vi "open.vi"(0 "object in":refnum<class "MBinteractive.lvclass">, 5 "error in (no error)":errorcluster) -> (14 "object out":refnum<class "MBinteractive.lvclass">, 19 "error out":errorcluster)   [LabVIEW 2016, in "MBinteractive.lvclass"]
uses:
  MBinteractive.lvclass
  <vilib>/NI/Modbus Library/API/Modbus API.lvclass/Modbus API.ctl
  <vilib>/NI/Modbus Library/Transmission Data Unit/Transmission Data Unit.lvclass/Transmission Data Unit.ctl
  MBinteractive.lvclass/MBinteractive.ctl
  <vilib>/NI/Modbus Library/API/Master/Set Unit ID.vi
  <vilib>/NI/Modbus Library/Transmission Data Unit/Write Unit ID.vi
  <vilib>/NI/Modbus Library/API/Read Transmission Data Unit.vi
  <vilib>/NI/Modbus Library/API/Write Transmission Data Unit.vi
  <vilib>/NI/Modbus Library/API/master/Modbus Master.lvclass
  D:/Program Files (x86)/National Instruments/LabVIEW 2016/vi.lib/NI/Modbus Library/API/Modbus API.lvclass
  <vilib>/NI/Modbus Library/API/Wrapper/Create TCP Master.vi
  <vilib>/NI/Modbus Library/API/Wrapper/API Main.lvlib
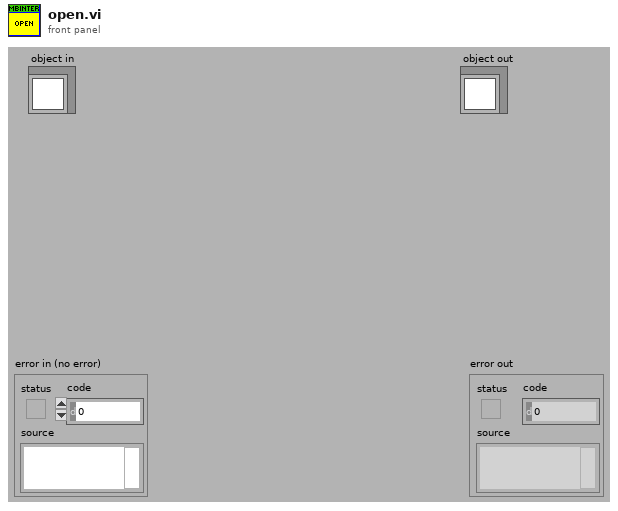
[diagram p1: front panel]
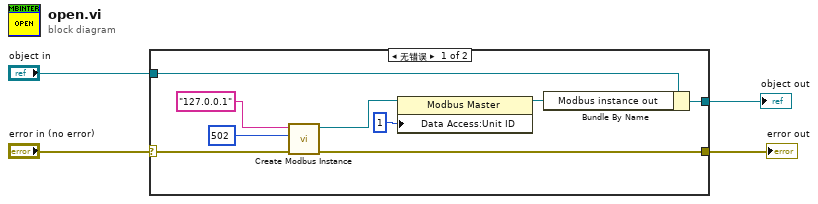
[diagram p0: block diagram]
diagram:
  n1 = case shown="无错误" "error in (no error)" {
    selector: "error in (no error)" -> [w6 w15]
    tunnel: [w5 w15] -> w3
    tunnel: [w12 w14] -> w1
    tunnel: "object in" -> [w13 w14]
    frame No Error {
      n2 = call-poly <vilib>:"Create Modbus Instance.vi"("error in"=w6, "port (502)"=u16 502, "address"="127.0.0.1") -> ("error out"=w5:errorcluster, "TCP master instance"=w11:refnum<class "Modbus Master.lvclass">)  [unwired: 7 in]
      n3 = property class="Modbus Master"(reference=w11, "Data Access:Unit ID"=u8 1 ("Unit ID")) -> (reference out=w7:refnum<class "Modbus Master.lvclass">)  [unwired: 1 in, 1 out]
      n4 = Bundle By Name(cluster=w13, "Modbus instance out"=w7) -> (w12:refnum<class "MBinteractive.lvclass">)
    }
    frame Error {
    }
  }
  "error out" <- w3
  "object out" <- w1
